vi "Write Name.vi"(8 "error in (no error)":errorcluster, 10 "Name":string, 11 "SQS in":refnum<class "SQS.lvclass">) -> (0 "error out":errorcluster, 3 "SQS out":refnum<class "SQS.lvclass">)   [LabVIEW 2015, in "NI_SQS.lvlib" / "SQS.lvclass"]
uses:
  SQS.lvclass
  SQS.lvclass/SQS.ctl
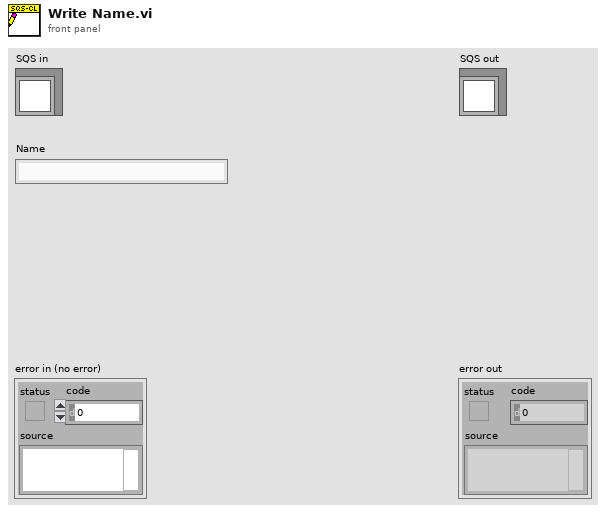
[diagram p1: front panel]
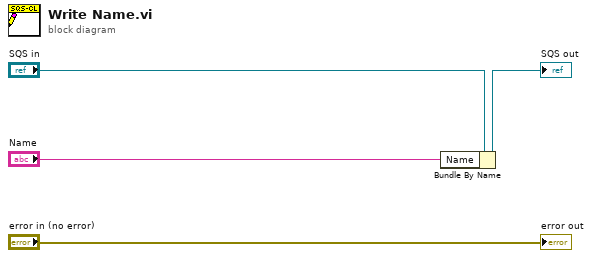
[diagram p0: block diagram]
diagram:
  n1 = Bundle By Name(cluster="SQS in", "Name"="Name") -> (→"SQS out":refnum<class "SQS.lvclass">)
  "error out" <- "error in (no error)"
